vi "Compute Orphaned Keys.vi"(9 "Registration Parent Keys":string[](array[string]), 10 "Registration Keys":string[](array[string]), 11 "Assert Parent Keys":string[](array[string])) -> (3 "Orphaned Registration Keys":string[](array[string]))   [LabVIEW 2020, in "Caraya.lvlib" / "Basic Test Manager.lvclass"]
uses:
  Basic Test Manager.lvclass
  Basic Test Manager.lvclass/Basic Test Manager.ctl
  <userlib>/_OpenG.lib/array/array.llb/openg_array.lvlib
  <userlib>/_OpenG.lib/array/array.llb/Remove Duplicates from 1D Array (I32)__ogtk.vi
  <userlib>/_OpenG.lib/array/array.llb/Delete Elements from 1D Array (String)__ogtk.vi
  <userlib>/_OpenG.lib/array/array.llb/Search 1D Array (String)__ogtk.vi
  <userlib>/_OpenG.lib/array/array.llb/Filter 1D Array (String)__ogtk.vi
  <userlib>/_OpenG.lib/array/array.llb/Empty 1D Array (String)__ogtk.vi
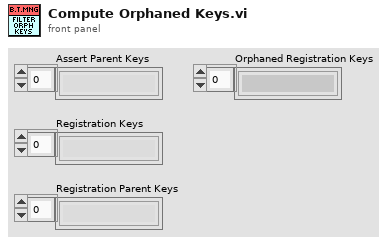
[diagram p1: front panel]
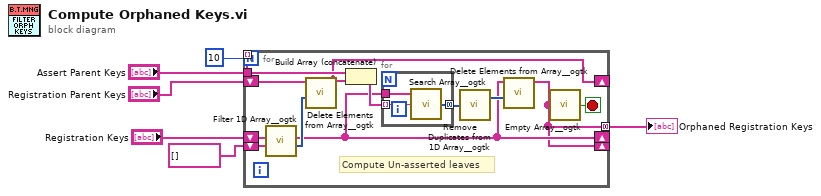
[diagram p0: block diagram]
diagram:
  n1 = for {
    N: 10 -> [_]
    tunnel: "Assert Parent Keys" -> [w14]
    shift-right: [w7] -> _
    shift-left: string[] [] ("array w/ subset deleted") -> [w16]
    tunnel: [w7] -> w6 mode=concatenating
    shift-right: [w9] -> _
    shift-left: "Registration Parent Keys" -> [w11]
    tunnel: [w14] -> _ mode=indexing
    shift-right: [w8] -> _
    shift-left: "Registration Keys" -> [w15]
    stop <- w12 stop-if-true
    # "Compute Un-asserted leaves"
    n2 = call-poly <userlib>:"Filter 1D Array__ogtk.vi"("items to filter"=w16, "array"=w15) -> ("filtered item indices"=w10:i32[], "filtered array"=w8:string[])  [unwired: 4 in]
    n3 = call-poly <userlib>:"Delete Elements from Array__ogtk.vi"("indices"=w10, "array"=w11) -> ("array w/ subset deleted"=w9:string[])  [unwired: 8 in, 1 out]
    n4 = Build Array (concatenate)(w14, w9) -> (w17:string[])
    n5 = for {
      tunnel: w8 -> [w21]
      tunnel: [w20] -> w18 mode=concatenating
      tunnel: w17 -> [w19] mode=indexing
      n6 = call-poly <userlib>:"Search Array__ogtk.vi"("Array"=w21, "Element Data"=w19) -> ("Indices of Elements"=w20:i32[])  [unwired: 7 in]
    }
    n7 = call-poly <userlib>:"Remove Duplicates from 1D Array__ogtk.vi"("Input Array"=w18) -> ("Output Array"=w13:i32[])  [unwired: 1 out]
    n8 = call-poly <userlib>:"Delete Elements from Array__ogtk.vi"("indices"=w13, "array"=w8) -> ("array w/ subset deleted"=w7:string[])  [unwired: 8 in, 1 out]
    n9 = call-poly <userlib>:"Empty Array__ogtk.vi"("Array"=w7) -> ("Empty Array?"=w12:bool)  [unwired: 8 in]
  }
  "Orphaned Registration Keys" <- w6
